vi "Untitled 1 (SubVI).vi"(8 "error in (no error)":errorcluster, 9 "Array in":i32[](array[numeric]), 10 "loop 1":i32, 11 "Refnum in":refnum<k35>) -> (0 "error out":errorcluster, 1 "Array 3":dbl[](array[numeric]), 2 "Array out":i32[](array[numeric]), 3 "Refnum out":refnum<k35>)   [LabVIEW 2021]
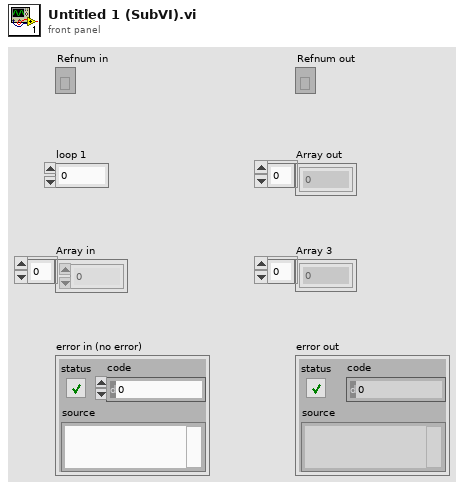
[diagram p1: front panel]
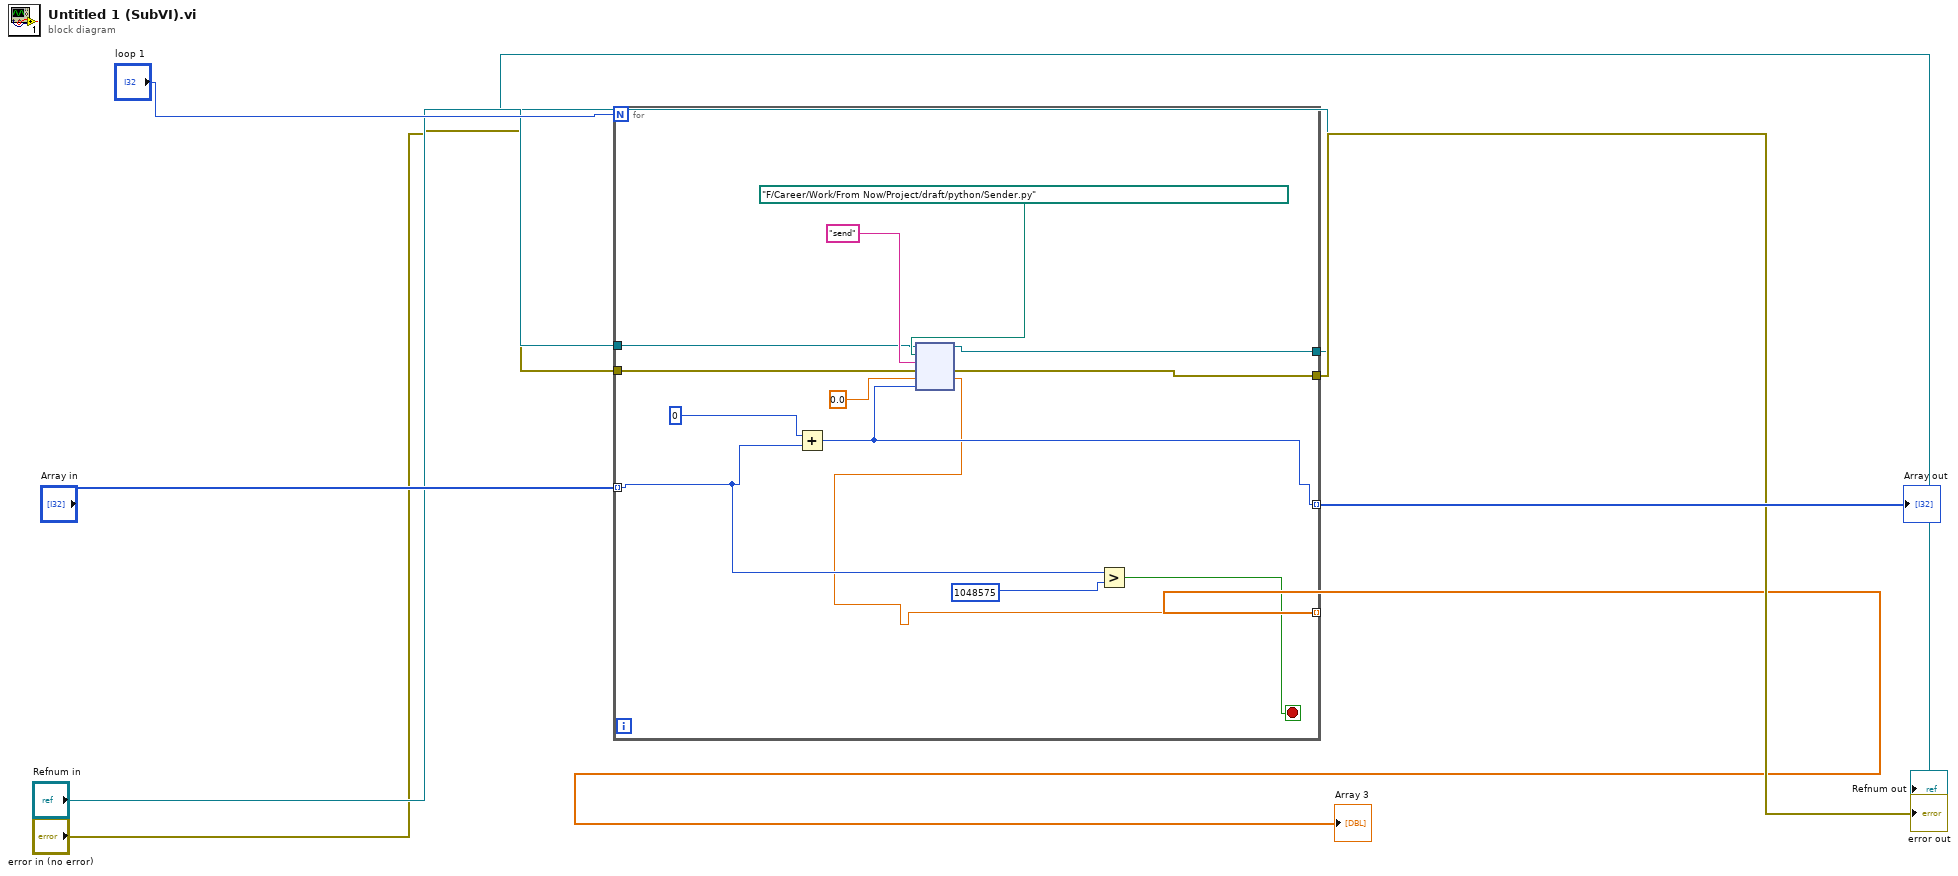
[diagram p0: block diagram]
diagram:
  n1 = for {
    N: "loop 1" -> [_]
    tunnel: [w9] -> w2 mode=indexing
    tunnel: [w19] -> w1
    tunnel: [w18] -> w3
    tunnel: "Refnum in" -> [w17]
    tunnel: "error in (no error)" -> [w16]
    tunnel: "Array in" -> [w11] mode=indexing
    tunnel: [w10] -> w8 mode=indexing
    stop <- w15 stop-if-true
    n2 = Add(x=0, y=w11) -> (x+y=w10:i32)
    n3 = node(w17, path "F:/Career/Work/From Now/Project/draft/python/Sender.py" ("module path"), "send" ("function name"), w16, 0.0, w10) -> (w19:refnum<k35>, w18:errorcluster, w9:dbl)  [unwired: 1 in, 2 out]
    n4 = Greater?(x=w11, y=1048575) -> (0:w15:bool)
  }
  "Array out" <- w8
  "error out" <- w3
  "Array 3" <- w2
  "Refnum out" <- w1
